vi "AcidClean.vi"() -> ()   [LabVIEW 2019]
uses:
  <vilib>/NI/Current Value Table/Type Defs/Single Tag.ctl
  <vilib>/NI/Current Value Table/Type Defs/Data Types.ctl
  <vilib>/Utility/miscctls.llb/LVPointTypeDef.ctl
  <vilib>/NI/STM/TCP/Read Meta Data (TCP Ref).vi
  <vilib>/NI/STM/TCP/Get Connection Reference (TCP).vi
  <vilib>/NI/AMC/Read Termination Message.vi
  <vilib>/NI/AMC/Create Single Message.vi
  <vilib>/NI/AMC/Update Message Routing Info.vi
  <vilib>/NI/STM/TCP/Read Meta Data (TCP Clst).vi
  <vilib>/NI/AMC/Globals.vi
  <vilib>/NI/STM/TCP/Write Message (TCP).vi
  <vilib>/NI/AMC/Send Message.vi
  <vilib>/NI/AMC/AMC.lvlib
  <vilib>/NI/STM/NI STM.lvlib
  <vilib>/NI/Current Value Table/Current Value Table.lvlib
panel:
  in  "AcidT3 Cntrl T Last Hr":bool
  out "Cleaner Control Temperature":dbl(slide) scale=0.0..60.0
  in  "Level Setpoint":dbl(knob)=40.0 min=40.0 max=85.0 step=0.5 scale=40.0..85.0
  in  "Enable Auto Fill":bool
  in  "AcidT3 Flow Last Hr":bool
  in  "AcidT3 Lev Last Hr":bool
  in  "AcidT3 T Last Hr":bool
  in  "Temperature Setpoint":dbl(knob)=25.0 min=20.0 max=60.0 step=0.5 scale=20.0..60.0
  in  "Enable Heat":bool
  out "Heater 2":bool
  out "Boolean 4":bool
  out "Boolean 2":bool
  out "Boolean 5":bool
  out "Drain":bool
  out "SuckPipe 2":bool
  out "Main Pump":bool
  in  "Tab Control":enum32{"Page 1", "ENG"}(tab)
  out "Heater Enabled":bool
  out "Amps":dbl format="%#.2g"
  out "Volts":dbl format="%#.1f"
  out "VFD T":dbl format="%#.2g"
  out "RPM":dbl format="%#.0f"
  out "Fault Code":dbl format="%#.2g"
  out "Freq":dbl format="%#.2g"
  in  "Drain Acid Clean":bool
  out "Level (L)":dbl(slide) scale=0.0..100.0
  in  "Specific Gravity":dbl(knob)=1.0 min=1.0 max=1.3 step=0.0025 scale=1.0..1.3
  out "E Stop":bool
  out "Run Enabled?":bool
  out "Cleaner Tank Temperature":dbl(slide) scale=0.0..60.0
  in  "Flow Setpoint":dbl(knob)=25.0 min=25.0 max=100.0 step=1.0 scale=25.0..100.0
  in  "Enable Clean":bool
  out "Flow rate":dbl(knob) scale=0.0..100.0
  in  "Machine":bool
  in  "Basement 4":bool
  in  "Dryer":bool
  in  "Rinse 4":bool
  in  "Rinse 3":bool
  in  "Rinse 2":bool
  in  "Basement 3":bool
  in  "Basement 2":bool
  in  "Basement 1":bool
  in  "Plater 6":bool
  in  "Plater 5":bool
  in  "Plater 4":bool
  in  "Plater 3":bool
  in  "Plater 2":bool
  in  "Plater 1":bool
  in  "Predip":bool
  in  "Rinse 1":bool
  in  "Cleaner":bool
  in  "Etch":bool
  out "status":string
  # "Module Selection"
  # "L/min"
  # "°C"
  # "°C"
  # "Motor Parameters"
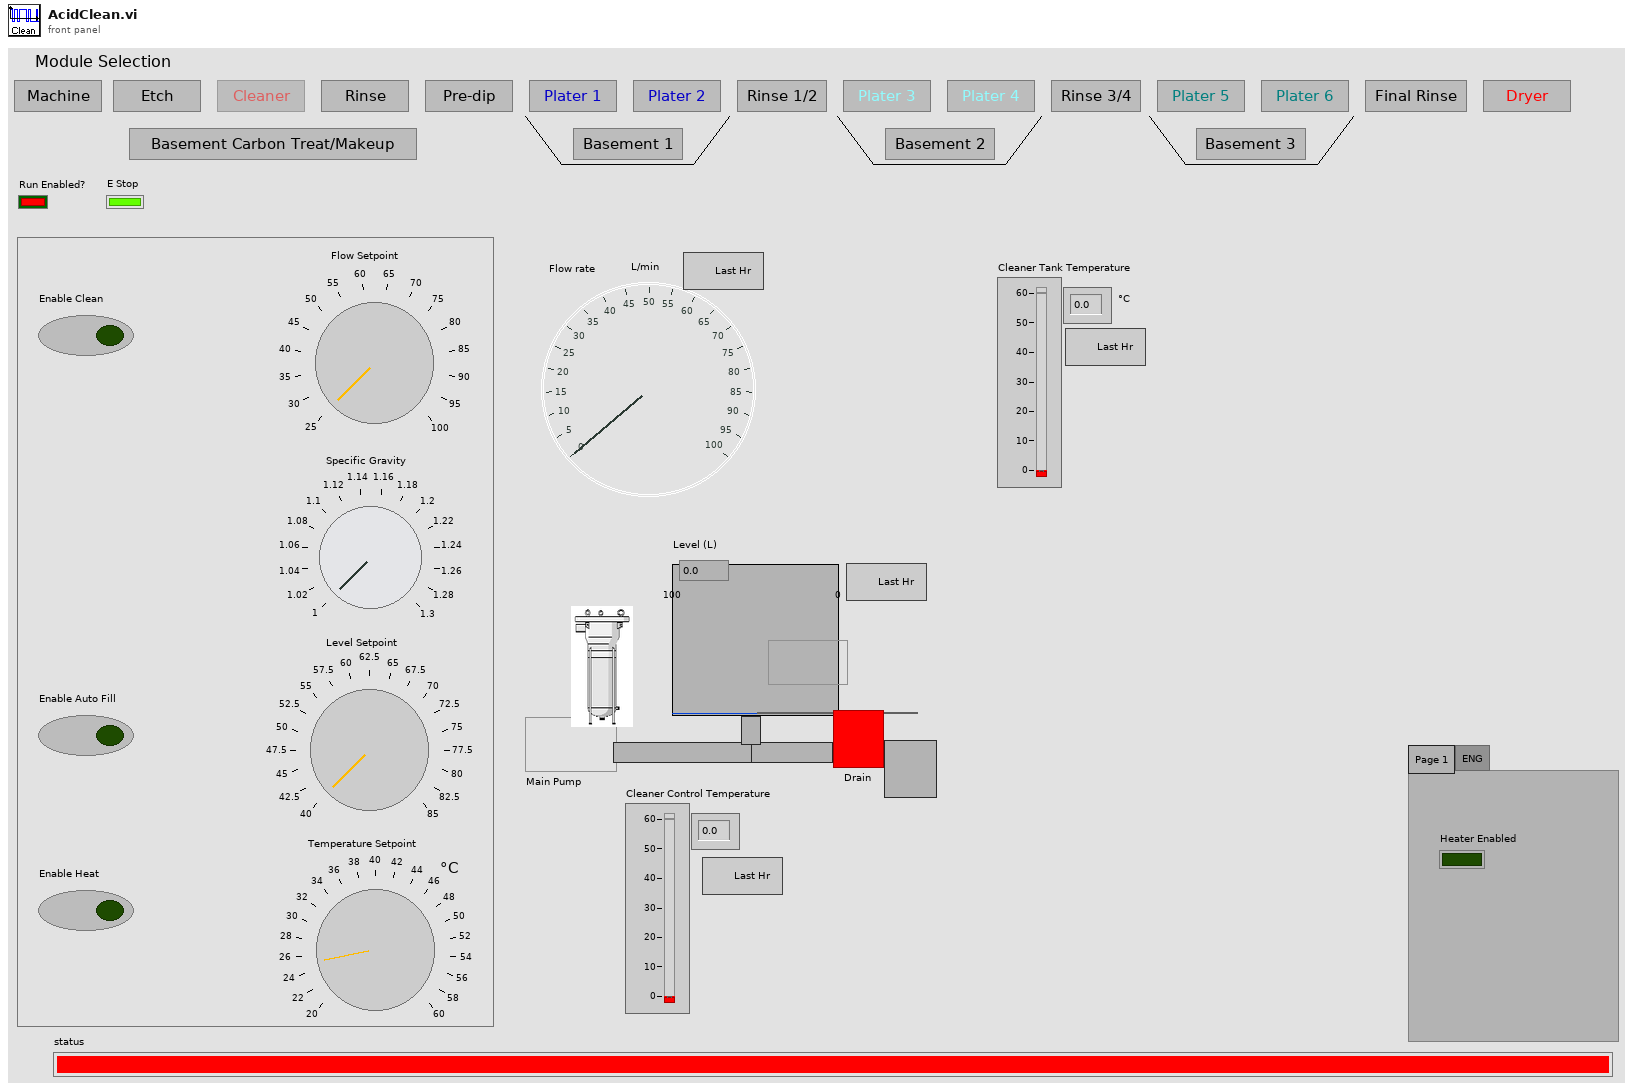
[diagram p1: front panel]
types:
  T1 = typedef "Current Value Table.lvlib/Single Tag.ctl" = cluster{"Data Type":T2, "Name":string, "Value":string, "Description":string}
  T2 = typedef "Current Value Table.lvlib/Data Types.ctl" = enum16{"Double", "Single", "I64", "I32", "I16", "I8", "U64", "U32", "U16", "U8", "String", "Boolean", "Array of U8", "Array of U16", "Array of U32", "Array of U64", "Array of I64", "Array of I32", "Array of I16", "Array of I8", "Array of Double", "Array of Single", "Array of Boolean", "Array of String"}
  T3 = typedef "NI STM.lvlib/TCP Connection Info.ctl" = cluster{"connection ID":refnum<k5>, "meta data":T4[]}
  T4 = typedef "NI STM.lvlib/MetaDataElement.ctl" = string
  T5 = typedef "AMC.lvlib/Message Queue.ctl" = refnum<queue>
  T6 = cluster{"Shift":bool, "Ctrl":bool, "Alt":bool, "Cmd":bool, "Opt":bool}
  T7 = typedef "LVPointTypeDef.ctl" = cluster{"Horizontal":i16, "Vertical":i16}
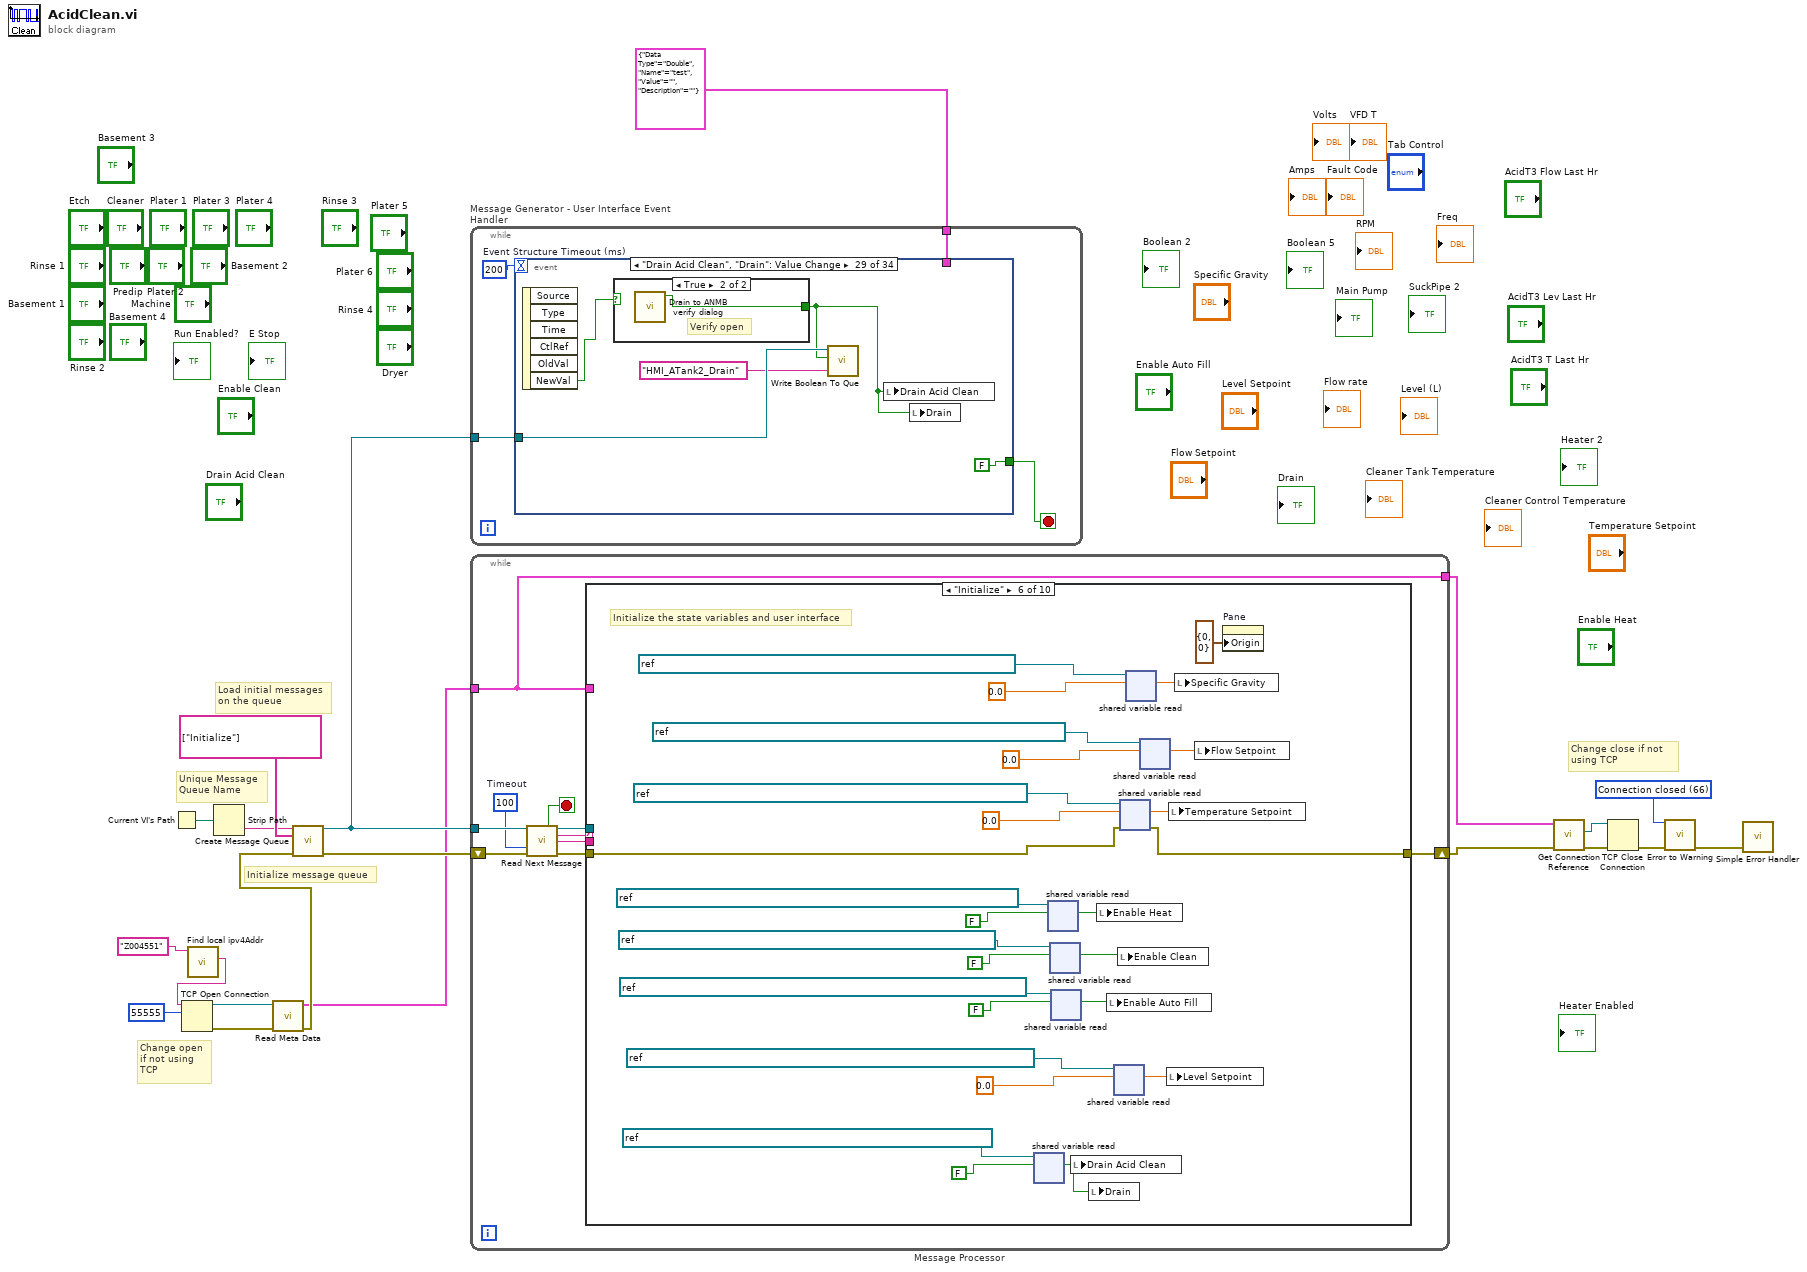
[diagram p0: block diagram]
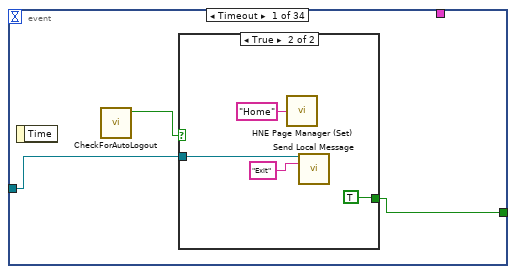
[diagram p2: hidden frame]
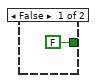
[diagram p3: hidden frame]
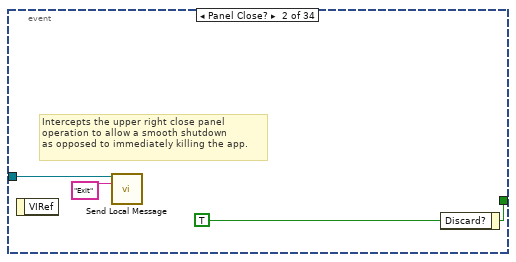
[diagram p4: hidden frame]
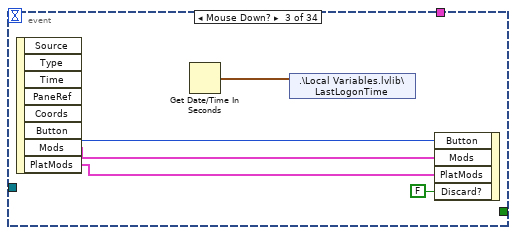
[diagram p5: hidden frame]
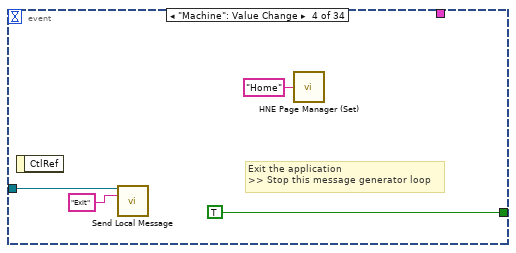
[diagram p6: hidden frame]
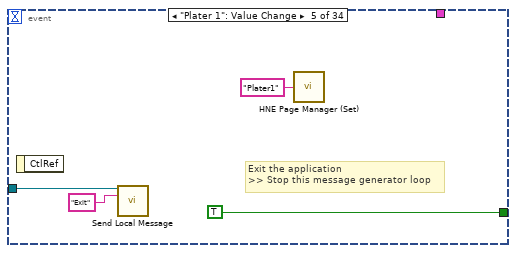
[diagram p7: hidden frame]
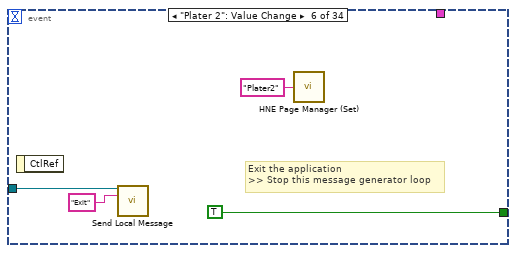
[diagram p8: hidden frame]
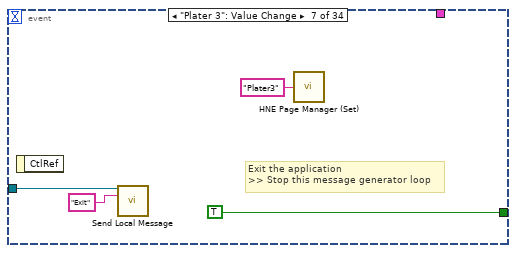
[diagram p9: hidden frame]
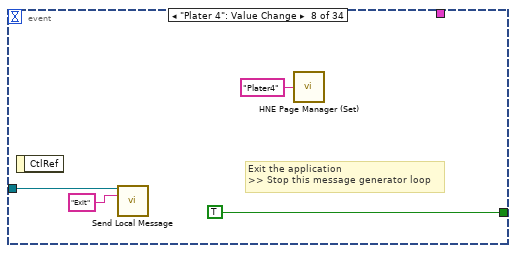
[diagram p10: hidden frame]
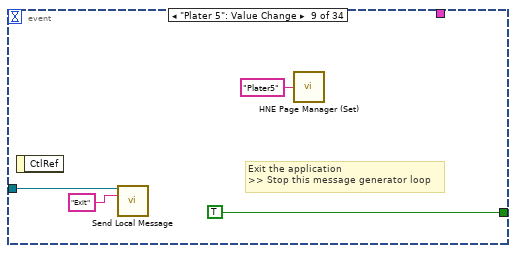
[diagram p11: hidden frame]
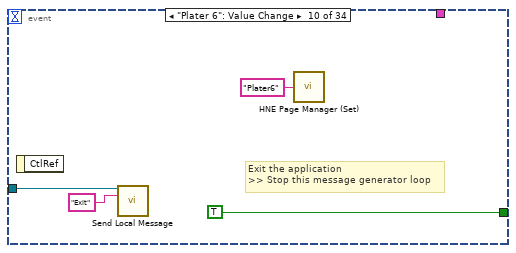
[diagram p12: hidden frame]
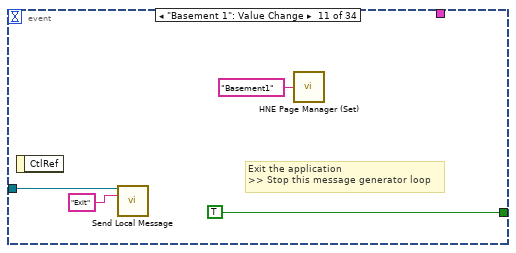
[diagram p13: hidden frame]
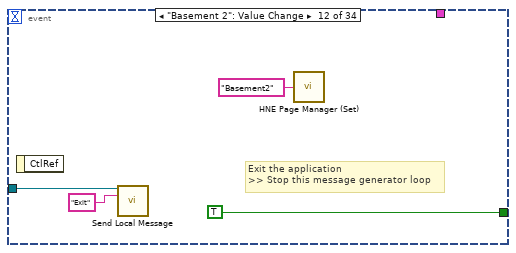
[diagram p14: hidden frame]
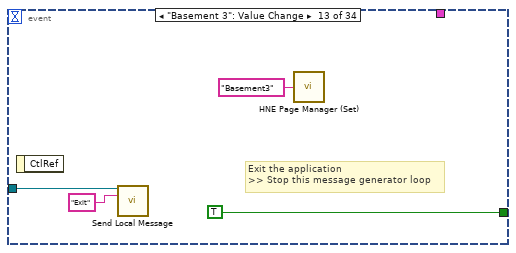
[diagram p15: hidden frame]
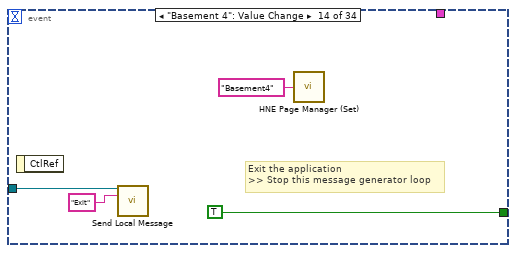
[diagram p16: hidden frame]
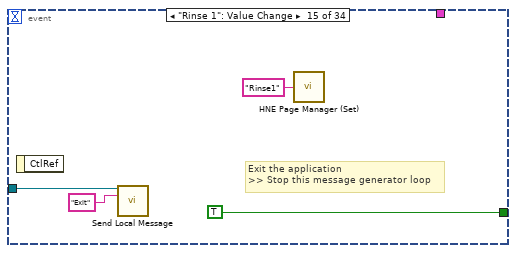
[diagram p17: hidden frame]
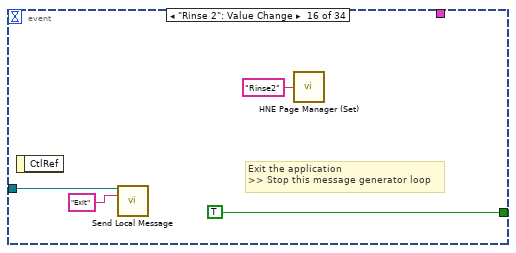
[diagram p18: hidden frame]
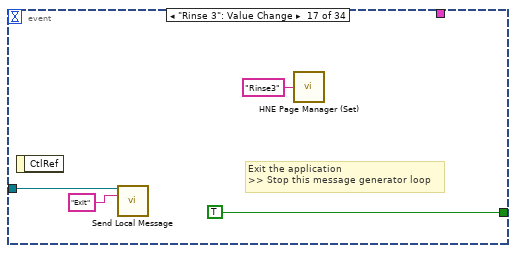
[diagram p19: hidden frame]
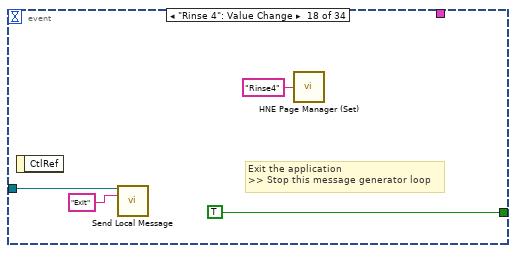
[diagram p20: hidden frame]
diagram:
  w9 = 66 items=["No Error", "Argument Error", "Memory Full", "Out of Zone", "End of File", "File Already Open", "Generic File IO Error", "File Not Found", "File Permission Error", "Disk Full", "Duplicate Path", "Too Many Files Open", "Not Enabled", "Resource File Not Found", "Cannot Add Resource", "Resource Not Found", "Image Not Found", "Image Memory Error", "Pen Does Not Exist", "Config Bad Type", "Config Token Not Found", "Config Parse Error", "Config Memory Error", "Bad External Code Format", "Bad External Code Offset", "External Code Not Present", "Null Window", "Destroy Window Mixup", "Null Menu", "Print Aborted", "Bad Print Record", "Print Driver Error", "Windows Error During Print", "Memory Error During Print", "Print Dialog Error", "Generic Print Error", "Invalid Device Refnum", "Device Not Found", "Device Parameter Error", "Device Unit Error", "Can't Open Device", "Device Call Aborted", "Generic Error", "Cancelled By User", "Object ID Too Low", "Object ID Too High", "Object Not In Heap", "Unknown Heap", "Bad DefProc ID", "DefProc Not In Table", "Message Out Of Range", "Null Method", "Unknown Message", "Manager Call Not Supported", "Bad address", "Connection In progress", "Connection timed out", "Connection is already in progress", "Network attribute not supported", "Network error", "Address in use", "System out of memory", "Connection aborted", "Connection refused", "Connection is not connected", "Connection is already connected", "Connection closed", "Initialize error (interapplication manager)", "Bad occurrence", "Wait on unbound occurrence handler", "Occurrence queue overflow", "Bad path", "Semaphore not signaled", "Unrecognized type (interapplication manager)"] ("1st Error to Convert")
  # "Change close if not using TCP"
  # "Change open if not using TCP"
  # "Initialize message queue"
  # "Unique Message\nQueue Name"
  # "Load initial messages\non the queue"
  n1 = Current VI's Path() -> (path=w16:path)
  n2 = call "Find local ipv4Addr.vi"("MachineToFind"="Z004551" ("Target IP Address")) -> ("name"=w2:string)  [unwired: 9 in, 1 out]
  n3 = TCP Open Connection(address=w2, remote port or service name=u16 55555 ("remote port")) -> (connection ID=w14:refnum<k5>, error out=w13:errorcluster)  [unwired: 1 in, 2 out]
  n4 = Strip Path(path=w16) -> (name=w19:string)  [unwired: 1 out]
  n5 = call-poly <vilib>:"Read Meta Data.vi"("error in"=w13, "connection ID"=w14) -> ("error out"=w12:errorcluster, "connection info out"=w11:T3)  [unwired: 7 in, 1 out]
  n6 = call <vilib>:"Create Message Queue.vi"("message queue name"=w19, "initial message names"=string[] ["Initialize"], "error in"=w12) -> ("message queue out"=w18:T5, "error out"=w17:errorcluster)  [unwired: 11 in]
  n7 = while "Message Generator - User Interface Event Handler" {
    tunnel: w18 -> [w22]
    tunnel: T1 {"Data Type"=enum."Double", "Name"="test", "Value"="", "Description"=""} ("Tag") -> [w21]
    stop <- w23 stop-if-true
    w24 = 200  # Event Structure Timeout (ms)
    n8 = event shown="[28] \"Drain Acid Clean\", \"Drain\": Value Change" {
      selector: _ -> [_ _ _ _ _ _ _ _ _ _ _ _ _ _ _ _ _ _ _ _ _ _ _ _ _ _ _ _ _ _ _ _ _ _]
      dyn-events: _ -> [_ _ _ _ _ _ _ _ _ _ _ _ _ _ _ _ _ _ _ _ _ _ _ _ _ _ _ _ _ _ _ _ _ _]
      timeout: w24 -> [_ _ _ _ _ _ _ _ _ _ _ _ _ _ _ _ _ _ _ _ _ _ _ _ _ _ _ _ _ _ _ _ _ _]
      tunnel: [w25 w35 _ TRUE ("Discard?") TRUE ("Discard?") TRUE ("Discard?") TRUE ("Discard?") TRUE ("Discard?") TRUE ("Discard?") TRUE ("Discard?") TRUE ("Discard?") TRUE ("Discard?") TRUE ("Discard?") TRUE ("Discard?") TRUE ("Discard?") TRUE ("Discard?") TRUE ("Discard?") TRUE ("Discard?") TRUE ("Discard?") TRUE ("Discard?") TRUE ("Discard?") FALSE ("Discard?") FALSE ("Discard?") FALSE ("Discard?") _ _ _ _ FALSE ("Discard?") FALSE ("Discard?") FALSE ("Discard?") FALSE ("Discard?") FALSE ("Discard?") _] -> w23
      tunnel: w22 -> [w26 w33 _ w42 w46 w50 w54 w58 w62 w66 w70 w74 w78 w82 w86 w90 w94 w98 w102 w106 w110 w121 w132 w143 w146 w151 w156 w161 w169 w180 w190 w200 w210 w213]
      tunnel: w21 -> [_ _ _ _ _ _ _ _ _ _ _ _ _ _ _ _ _ _ _ _ _ w115 w126 w137 _ _ _ _ _ w176 w186 w196 w206 _]
      event Timeout {
        n9 = event-data() -> ()  [unwired: 2 out]
        n10 = call "CheckForAutoLogout.vi"() -> ("Boolean"=w27:bool)  [unwired: 11 in]
        n11 = case shown="True" w27 {
          tunnel: [FALSE ("Discard?") TRUE ("Discard?")] -> w25
          tunnel: w26 -> [_ w29]
          frame False {
          }
          frame True {
            n12 = call <userlib>:"HNE Page Manager (Set).vi"("Next Page"="Home") -> ()  [unwired: 4 in, 1 out]
            n13 = call <vilib>:"Send Local Message.vi"("message queue in"=w29, "message name"="Exit") -> ()  [unwired: 11 in, 3 out]
          }
        }
      }
      event Panel Close? {
        w35 = TRUE ("Discard?")
        # "Intercepts the upper right close panel\noperation to allow a smooth shutdown\nas opposed to immediately killing the app."
        n14 = event-data() -> ()  [unwired: 2 out]
        n15 = call <vilib>:"Send Local Message.vi"("message queue in"=w33, "message name"="Exit") -> ()  [unwired: 11 in, 3 out]
        n16 = event-data("Discard?"=w35) -> ()  [unwired: 1 in, 1 out]
      }
      event Mouse Down? {
        n17 = event-data() -> ("Button"=w39:u16, "Mods"=w38:cluster{"Double Click":bool, "Menu Key":bool}, "PlatMods"=w37:T6)  [unwired: 6 out]
        n18 = Get Date/Time In Seconds() -> (seconds since 1Jan1904=w36:timestamp)
        n19 = shared-variable ".\\Local Variables.lvlib\\LastLogonTime"(w36) -> ()  [unwired: 1 in, 1 out]
        n20 = event-data("Button"=w39, "Mods"=w38, "PlatMods"=w37, "Discard?"=FALSE) -> ()  [unwired: 1 in, 1 out]
      }
      event "Machine": Value Change {
        # "Exit the application\n>> Stop this message generator loop"
        n21 = event-data() -> ()  [unwired: 2 out]
        n22 = call <vilib>:"Send Local Message.vi"("message queue in"=w42, "message name"="Exit") -> ()  [unwired: 11 in, 3 out]
        n23 = call <userlib>:"HNE Page Manager (Set).vi"("Next Page"="Home") -> ()  [unwired: 4 in, 1 out]
      }
      event "Plater 1": Value Change {
        # "Exit the application\n>> Stop this message generator loop"
        n24 = event-data() -> ()  [unwired: 2 out]
        n25 = call <vilib>:"Send Local Message.vi"("message queue in"=w46, "message name"="Exit") -> ()  [unwired: 11 in, 3 out]
        n26 = call <userlib>:"HNE Page Manager (Set).vi"("Next Page"="Plater1") -> ()  [unwired: 4 in, 1 out]
      }
      event "Plater 2": Value Change {
        # "Exit the application\n>> Stop this message generator loop"
        n27 = event-data() -> ()  [unwired: 2 out]
        n28 = call <vilib>:"Send Local Message.vi"("message queue in"=w50, "message name"="Exit") -> ()  [unwired: 11 in, 3 out]
        n29 = call <userlib>:"HNE Page Manager (Set).vi"("Next Page"="Plater2") -> ()  [unwired: 4 in, 1 out]
      }
      event "Plater 3": Value Change {
        # "Exit the application\n>> Stop this message generator loop"
        n30 = event-data() -> ()  [unwired: 2 out]
        n31 = call <vilib>:"Send Local Message.vi"("message queue in"=w54, "message name"="Exit") -> ()  [unwired: 11 in, 3 out]
        n32 = call <userlib>:"HNE Page Manager (Set).vi"("Next Page"="Plater3") -> ()  [unwired: 4 in, 1 out]
      }
      event "Plater 4": Value Change {
        # "Exit the application\n>> Stop this message generator loop"
        n33 = event-data() -> ()  [unwired: 2 out]
        n34 = call <vilib>:"Send Local Message.vi"("message queue in"=w58, "message name"="Exit") -> ()  [unwired: 11 in, 3 out]
        n35 = call <userlib>:"HNE Page Manager (Set).vi"("Next Page"="Plater4") -> ()  [unwired: 4 in, 1 out]
      }
      event "Plater 5": Value Change {
        # "Exit the application\n>> Stop this message generator loop"
        n36 = event-data() -> ()  [unwired: 2 out]
        n37 = call <vilib>:"Send Local Message.vi"("message queue in"=w62, "message name"="Exit") -> ()  [unwired: 11 in, 3 out]
        n38 = call <userlib>:"HNE Page Manager (Set).vi"("Next Page"="Plater5") -> ()  [unwired: 4 in, 1 out]
      }
      event "Plater 6": Value Change {
        # "Exit the application\n>> Stop this message generator loop"
        n39 = event-data() -> ()  [unwired: 2 out]
        n40 = call <vilib>:"Send Local Message.vi"("message queue in"=w66, "message name"="Exit") -> ()  [unwired: 11 in, 3 out]
        n41 = call <userlib>:"HNE Page Manager (Set).vi"("Next Page"="Plater6") -> ()  [unwired: 4 in, 1 out]
      }
      event "Basement 1": Value Change {
        # "Exit the application\n>> Stop this message generator loop"
        n42 = event-data() -> ()  [unwired: 2 out]
        n43 = call <vilib>:"Send Local Message.vi"("message queue in"=w70, "message name"="Exit") -> ()  [unwired: 11 in, 3 out]
        n44 = call <userlib>:"HNE Page Manager (Set).vi"("Next Page"="Basement1") -> ()  [unwired: 4 in, 1 out]
      }
      event "Basement 2": Value Change {
        # "Exit the application\n>> Stop this message generator loop"
        n45 = event-data() -> ()  [unwired: 2 out]
        n46 = call <vilib>:"Send Local Message.vi"("message queue in"=w74, "message name"="Exit") -> ()  [unwired: 11 in, 3 out]
        n47 = call <userlib>:"HNE Page Manager (Set).vi"("Next Page"="Basement2") -> ()  [unwired: 4 in, 1 out]
      }
      event "Basement 3": Value Change {
        # "Exit the application\n>> Stop this message generator loop"
        n48 = event-data() -> ()  [unwired: 2 out]
        n49 = call <vilib>:"Send Local Message.vi"("message queue in"=w78, "message name"="Exit") -> ()  [unwired: 11 in, 3 out]
        n50 = call <userlib>:"HNE Page Manager (Set).vi"("Next Page"="Basement3") -> ()  [unwired: 4 in, 1 out]
      }
      event "Basement 4": Value Change {
        # "Exit the application\n>> Stop this message generator loop"
        n51 = event-data() -> ()  [unwired: 2 out]
        n52 = call <vilib>:"Send Local Message.vi"("message queue in"=w82, "message name"="Exit") -> ()  [unwired: 11 in, 3 out]
        n53 = call <userlib>:"HNE Page Manager (Set).vi"("Next Page"="Basement4") -> ()  [unwired: 4 in, 1 out]
      }
      event "Rinse 1": Value Change {
        # "Exit the application\n>> Stop this message generator loop"
        n54 = event-data() -> ()  [unwired: 2 out]
        n55 = call <vilib>:"Send Local Message.vi"("message queue in"=w86, "message name"="Exit") -> ()  [unwired: 11 in, 3 out]
        n56 = call <userlib>:"HNE Page Manager (Set).vi"("Next Page"="Rinse1") -> ()  [unwired: 4 in, 1 out]
      }
      event "Rinse 2": Value Change {
        # "Exit the application\n>> Stop this message generator loop"
        n57 = event-data() -> ()  [unwired: 2 out]
        n58 = call <vilib>:"Send Local Message.vi"("message queue in"=w90, "message name"="Exit") -> ()  [unwired: 11 in, 3 out]
        n59 = call <userlib>:"HNE Page Manager (Set).vi"("Next Page"="Rinse2") -> ()  [unwired: 4 in, 1 out]
      }
      event "Rinse 3": Value Change {
        # "Exit the application\n>> Stop this message generator loop"
        n60 = event-data() -> ()  [unwired: 2 out]
        n61 = call <vilib>:"Send Local Message.vi"("message queue in"=w94, "message name"="Exit") -> ()  [unwired: 11 in, 3 out]
        n62 = call <userlib>:"HNE Page Manager (Set).vi"("Next Page"="Rinse3") -> ()  [unwired: 4 in, 1 out]
      }
      event "Rinse 4": Value Change {
        # "Exit the application\n>> Stop this message generator loop"
        n63 = event-data() -> ()  [unwired: 2 out]
        n64 = call <vilib>:"Send Local Message.vi"("message queue in"=w98, "message name"="Exit") -> ()  [unwired: 11 in, 3 out]
        n65 = call <userlib>:"HNE Page Manager (Set).vi"("Next Page"="Rinse4") -> ()  [unwired: 4 in, 1 out]
      }
      event "Predip": Value Change {
        # "Exit the application\n>> Stop this message generator loop"
        n66 = event-data() -> ()  [unwired: 2 out]
        n67 = call <vilib>:"Send Local Message.vi"("message queue in"=w102, "message name"="Exit") -> ()  [unwired: 11 in, 3 out]
        n68 = call <userlib>:"HNE Page Manager (Set).vi"("Next Page"="Predip") -> ()  [unwired: 4 in, 1 out]
      }
      event "Etch": Value Change {
        # "Exit the application\n>> Stop this message generator loop"
        n69 = event-data() -> ()  [unwired: 2 out]
        n70 = call <vilib>:"Send Local Message.vi"("message queue in"=w106, "message name"="Exit") -> ()  [unwired: 11 in, 3 out]
        n71 = call <userlib>:"HNE Page Manager (Set).vi"("Next Page"="Etch") -> ()  [unwired: 4 in, 1 out]
      }
      event "Dryer": Value Change {
        # "Exit the application\n>> Stop this message generator loop"
        n72 = event-data() -> ()  [unwired: 2 out]
        n73 = call <vilib>:"Send Local Message.vi"("message queue in"=w110, "message name"="Exit") -> ()  [unwired: 11 in, 3 out]
        n74 = call <userlib>:"HNE Page Manager (Set).vi"("Next Page"="Dryer") -> ()  [unwired: 4 in, 1 out]
      }
      event "Enable Clean": Value Change {
        n75 = event-data() -> ("NewVal"=w120:bool)  [unwired: 6 out]
        n76 = Boolean To (0,1)(Boolean=w120) -> (0, 1=w119:i16)
        n77 = Number To Decimal String(number=w119) -> (decimal integer string=w114:string)  [unwired: 1 in]
        n78 = Bundle By Name(cluster=w115, "Data Type"=Data_Types."Boolean", "Name"="HMI_ATank2_Enable", "Value"=w114) -> (w116:T1)
        n79 = Flatten To String(anything=w116) -> (data string=w113:string)  [unwired: 3 in, 2 out]
        n80 = call <vilib>:"Send Local Message.vi"("message queue in"=w121, "message name"="Write_Tag", "message value"=w113) -> ()  [unwired: 10 in, 3 out]
      }
      event "Enable Heat": Value Change {
        n81 = event-data() -> ("NewVal"=w131:bool)  [unwired: 6 out]
        n82 = Boolean To (0,1)(Boolean=w131) -> (0, 1=w130:i16)
        n83 = Number To Decimal String(number=w130) -> (decimal integer string=w125:string)  [unwired: 1 in]
        n84 = Bundle By Name(cluster=w126, "Data Type"=Data_Types."Boolean", "Name"="HMI_ATank2_HeatEnable", "Value"=w125) -> (w127:T1)
        n85 = Flatten To String(anything=w127) -> (data string=w124:string)  [unwired: 3 in, 2 out]
        n86 = call <vilib>:"Send Local Message.vi"("message queue in"=w132, "message name"="Write_Tag", "message value"=w124) -> ()  [unwired: 10 in, 3 out]
      }
      event "Enable Auto Fill": Value Change {
        n87 = event-data() -> ("NewVal"=w142:bool)  [unwired: 6 out]
        n88 = Boolean To (0,1)(Boolean=w142) -> (0, 1=w141:i16)
        n89 = Number To Decimal String(number=w141) -> (decimal integer string=w136:string)  [unwired: 1 in]
        n90 = Bundle By Name(cluster=w137, "Data Type"=Data_Types."Boolean", "Name"="HMI_ATank2_Fill_To_Level", "Value"=w136) -> (w138:T1)
        n91 = Flatten To String(anything=w138) -> (data string=w135:string)  [unwired: 3 in, 2 out]
        n92 = call <vilib>:"Send Local Message.vi"("message queue in"=w143, "message name"="Write_Tag", "message value"=w135) -> ()  [unwired: 10 in, 3 out]
      }
      event "AcidT3 Cntrl T Last Hr": Value Change {
        n93 = event-data() -> ("NewVal"=w147:bool)  [unwired: 6 out]
        n94 = case shown="True" w147 {
          tunnel: w146 -> [_ w150]
          frame False {
          }
          frame True {
            n95 = call <vilib>:"Send Local Message.vi"("message queue in"=w150, "message name"="DisplayLastHr", "message value"="Acid2_Temperature") -> ()  [unwired: 10 in, 3 out]
          }
        }
      }
      event "AcidT3 T Last Hr": Value Change {
        n96 = event-data() -> ("NewVal"=w152:bool)  [unwired: 6 out]
        n97 = case shown="True" w152 {
          tunnel: w151 -> [_ w155]
          frame False {
          }
          frame True {
            n98 = call <vilib>:"Send Local Message.vi"("message queue in"=w155, "message name"="DisplayLastHr", "message value"="AcidTnk2_Tank_T") -> ()  [unwired: 10 in, 3 out]
          }
        }
      }
      event "AcidT3 Lev Last Hr": Value Change {
        n99 = event-data() -> ("NewVal"=w157:bool)  [unwired: 6 out]
        n100 = case shown="True" w157 {
          tunnel: w156 -> [_ w160]
          frame False {
          }
          frame True {
            n101 = call <vilib>:"Send Local Message.vi"("message queue in"=w160, "message name"="DisplayLastHr", "message value"="Acid2_Level") -> ()  [unwired: 10 in, 3 out]
          }
        }
      }
      event "AcidT3 Flow Last Hr": Value Change {
        n102 = event-data() -> ("NewVal"=w162:bool)  [unwired: 6 out]
        n103 = case shown="True" w162 {
          tunnel: w161 -> [_ w165]
          frame False {
          }
          frame True {
            n104 = call <vilib>:"Send Local Message.vi"("message queue in"=w165, "message name"="DisplayLastHr", "message value"="Acid2_Flow") -> ()  [unwired: 10 in, 3 out]
          }
        }
      }
      event "Drain Acid Clean", "Drain": Value Change {
        n105 = event-data() -> ("NewVal"=w167:bool)  [unwired: 6 out]
        n106 = case shown="True" w167 {
          selector: w167 -> [w171 _]
          tunnel: [w171 w172] -> w166
          frame False {
            # "Always close"
          }
          frame True {
            # "Verify open"
            n107 = call "Drain to ANMB verify dialog.vi"() -> ("Drain?"=w172:bool)  [unwired: 11 in]
          }
        }
        n108 = call "Write Boolean To Que.vi"("Tag"="HMI_ATank2_Drain", "NewVal"=w166, "Queue in"=w169) -> ()  [unwired: 9 in]
        n109 = local write "Drain Acid Clean"(w166) -> ()
        n110 = local write "Drain"(w166) -> ()
      }
      event "Flow Setpoint": Value Change {
        n111 = event-data() -> ("NewVal"=w174:dbl)  [unwired: 6 out]
        n112 = Number To Fractional String(number=w174) -> (F-format string=w173:string)  [unwired: 3 in]
        n113 = Bundle By Name(cluster=w176, "Data Type"=Data_Types."Double", "Name"="HMI_ATNK2_Flow_Setpoint", "Value"=w173) -> (w177:T1)
        n114 = Flatten To String(anything=w177) -> (data string=w175:string)  [unwired: 3 in, 2 out]
        n115 = call <vilib>:"Send Local Message.vi"("message queue in"=w180, "message name"="Write_Tag", "message value"=w175) -> ()  [unwired: 10 in, 3 out]
      }
      event "Specific Gravity": Value Change {
        n116 = event-data() -> ("NewVal"=w184:dbl)  [unwired: 6 out]
        n117 = Number To Fractional String(number=w184) -> (F-format string=w183:string)  [unwired: 3 in]
        n118 = Bundle By Name(cluster=w186, "Data Type"=Data_Types."Double", "Name"="HMI_Acid2_Tank_SG", "Value"=w183) -> (w187:T1)
        n119 = Flatten To String(anything=w187) -> (data string=w185:string)  [unwired: 3 in, 2 out]
        n120 = call <vilib>:"Send Local Message.vi"("message queue in"=w190, "message name"="Write_Tag", "message value"=w185) -> ()  [unwired: 10 in, 3 out]
      }
      event "Temperature Setpoint": Value Change {
        n121 = event-data() -> ("NewVal"=w194:dbl)  [unwired: 6 out]
        n122 = Number To Fractional String(number=w194) -> (F-format string=w193:string)  [unwired: 3 in]
        n123 = Bundle By Name(cluster=w196, "Data Type"=Data_Types."Double", "Name"="HMI_ATNK2_T_Setpoint", "Value"=w193) -> (w197:T1)
        n124 = Flatten To String(anything=w197) -> (data string=w195:string)  [unwired: 3 in, 2 out]
        n125 = call <vilib>:"Send Local Message.vi"("message queue in"=w200, "message name"="Write_Tag", "message value"=w195) -> ()  [unwired: 10 in, 3 out]
      }
      event "Level Setpoint": Value Change {
        n126 = event-data() -> ("NewVal"=w204:dbl)  [unwired: 6 out]
        n127 = Number To Fractional String(number=w204) -> (F-format string=w203:string)  [unwired: 3 in]
        n128 = Bundle By Name(cluster=w206, "Data Type"=Data_Types."Double", "Name"="HMI_ATank2_Level_SetPnt", "Value"=w203) -> (w207:T1)
        n129 = Flatten To String(anything=w207) -> (data string=w205:string)  [unwired: 3 in, 2 out]
        n130 = call <vilib>:"Send Local Message.vi"("message queue in"=w210, "message name"="Write_Tag", "message value"=w205) -> ()  [unwired: 10 in, 3 out]
      }
      event Menu Selection (User) {
        # "Add run-time menu items to the message\nqueue. The message handler case names must match the menu ItemTag names."
        n131 = event-data() -> ("ItemTag"=w214:string)  [unwired: 1 out]
        n132 = call <vilib>:"Send Local Message.vi"("message queue in"=w213, "message name"=w214) -> ()  [unwired: 11 in, 3 out]
      }
    }
  }
  n133 = while "Message Processor" {
    shift-left: w17 -> [w220]
    shift-right: [w224] -> w4
    tunnel: w18 -> [w221]
    tunnel: w11 -> [w215]
    tunnel: [w215] -> w5
    stop <- w223 stop-if-true
    w216 = 100  # Timeout
    n134 = call <vilib>:"Read Next Message.vi"("message queue in"=w221, "timeout (1 ms)"=w216, "error in"=w220) -> ("exit process?"=w223:bool, "message queue out"=w222:T5, "message name"=w218:string, "message value"=w217:string, "error out"=w219:errorcluster)  [unwired: 5 in, 3 out]
    n135 = case shown="\"Initialize\"" w218 {
      selector: w218 -> [_ _ w233 _ _ _ _ _ _ _]
      tunnel: w222 -> [_ _ _ _ _ _ w266 _ _ _]
      tunnel: w219 -> [w225 w230 w234 w235 w237 w250 w267 w269 w273 w275]
      tunnel: [w225 w230 w234 errorcluster {"status"=FALSE, "code"=0, "source"=""} ("error out") w237 w249 w265 w269 w272 w275] -> w224
      tunnel: w217 -> [_ _ _ _ _ _ _ _ w270 w276]
      tunnel: w215 -> [_ _ _ _ _ _ _ _ w271 _]
      frame "---------- Framework Operations ----------" {
        # "Dummy case to add a seperator in the Case Structure menu"
      }
      frame "", "Idle" {
        # "Idle Case - this case is called after a Timeout on the Get Next Message from Queue VI, if no new messages are present on the queue. This case can be used for housekeeping tasks such as updating the UI."
        n136 = control-ref of="status"() -> (w229:refnum<vi>)
        n137 = local read "Main Pump"() -> (w227:bool)
        n138 = local read "Drain"() -> (w228:bool)
        n139 = call <userlib>:"TAE Format Alarm Ticker.vi"("Alarm Ticker Ref"=w229) -> ()  [unwired: 15 in]
        n140 = Or(x=w228, y=w227) -> (x .or. y?=→"Boolean 4":bool)
      }
      frame "Missing Message Handler", Default {
        # "Call this case if a message is received that is not handled \nby any other case. Typically this is a programming error\nas a result of a typo or unhandled message/missing message handler."
        n141 = Format Into String(format string="DevError: Missing message handler for '%s\" message." ("message"), w233) -> (resulting string=w231:string)  [unwired: 2 in, 1 out]
        n142 = One Button Dialog(message=w231) -> ()  [unwired: 2 out]
      }
      frame "Error" {
        # "General Error Case - this case is called if an error is passed using the error cluster below. Typically most new errors should be handed in each individual case and not passed in the rror cluster. If necessary a custom error handler case should be added and called from other cases."
        n143 = call <vilib>:"Simple Error Handler.vi"("error in (no error)"=w235) -> ()  [unwired: 1 in, 8 out]
      }
      frame "---------- Generic Operations ----------" {
        # "Dummy case to add a seperator in the Case Structure menu"
      }
      frame "Initialize" {
        # "Initialize the state variables and user interface"
        n144 = shared-variable-read(refnum<k21> "ni.var.psp://z004551/CDL0100 ReadWriteTags/HMI_ATank2_Drain" ("shared variable refnum in"), FALSE) -> (w253:bool)  [unwired: 1 in, 3 out]
        n145 = shared-variable-read(refnum<k21> "ni.var.psp://z004551/CDL0100 ReadWriteTags/HMI_ATank2_HeatEnable" ("shared variable refnum in"), FALSE) -> (w245:bool)  [unwired: 1 in, 3 out]
        n146 = shared-variable-read(refnum<k21> "ni.var.psp://z004551/CDL0100 ReadWriteTags/HMI_ATank2_Enable" ("shared variable refnum in"), FALSE) -> (w262:bool)  [unwired: 1 in, 3 out]
        n147 = shared-variable-read(refnum<k21> "ni.var.psp://z004551/CDL0100 ReadWriteTags/HMI_ATank2_Fill_To_Level" ("shared variable refnum in"), FALSE) -> (w242:bool)  [unwired: 1 in, 3 out]
        n148 = local write "Drain Acid Clean"(w253) -> ()
        n149 = local write "Drain"(w253) -> ()
        n150 = local write "Enable Heat"(w245) -> ()
        n151 = local write "Enable Auto Fill"(w242) -> ()
        n152 = shared-variable-read(refnum<k21> "ni.var.psp://z004551/CDL0100 ReadWriteTags/HMI_ATank2_Level_SetPnt" ("shared variable refnum in"), 0.0) -> (w239:dbl)  [unwired: 1 in, 3 out]
        n153 = local write "Enable Clean"(w262) -> ()
        n154 = shared-variable-read(refnum<k21> "ni.var.psp://z004551/CDL0100 ReadWriteTags/HMI_ATNK2_T_Setpoint" ("shared variable refnum in"), w250, 0.0) -> (w249:errorcluster, w248:dbl)  [unwired: 2 out]
        n155 = shared-variable-read(refnum<k21> "ni.var.psp://z004551/CDL0100 ReadWriteTags/HMI_Acid2_Tank_SG" ("shared variable refnum in"), 0.0) -> (w254:dbl)  [unwired: 1 in, 3 out]
        n156 = shared-variable-read(refnum<k21> "ni.var.psp://z004551/CDL0100 ReadWriteTags/HMI_ATNK2_Flow_Setpoint" ("shared variable refnum in"), 0.0) -> (w259:dbl)  [unwired: 1 in, 3 out]
        n157 = local write "Level Setpoint"(w239) -> ()
        n158 = local write "Temperature Setpoint"(w248) -> ()
        n159 = local write "Specific Gravity"(w254) -> ()
        n160 = local write "Flow Setpoint"(w259) -> ()
        n161 = property on="Pane" class="Pane"("Origin"=T7 {"Horizontal"=0, "Vertical"=0}) -> ()  [unwired: 2 in, 2 out]
      }
      frame "Exit" {
        # "Destroy message queue >> this will halt the UI event handler loop"
        # "Stop the VI\n>> Perform any cleanup tasks in this message case.\n>> Clear display before closing."
        n162 = call <vilib>:"Destroy Message Queue.vi"("message queue in"=w266, "error in"=w267) -> ("error out"=w265:errorcluster)  [unwired: 11 in, 2 out]
        n163 = local write "status"("" ("Status")) -> ()
      }
      frame "---------- Application Operations ----------" {
        # "Dummy case to add a seperator in the Case Structure menu"
      }
      frame "Write_Tag" {
        n164 = call-poly <vilib>:"Write Message.vi"("error in"=w273, "data"=w270, "name"="WriteTag", "connection info in"=w271) -> ("error out"=w272:errorcluster)  [unwired: 6 in, 1 out]
      }
      frame "DisplayLastHr" {
        n165 = call "Trace Variable 1 hour Popup.vi"("Tag"=w276) -> ()  [unwired: 11 in]
      }
    }
  }
  n166 = call-poly <vilib>:"Get Connection Reference.vi"("error in"=w4, "connection info in"=w5) -> ("error out"=w8:errorcluster, "connection ID out"=w7:refnum<k5>)  [unwired: 8 out]
  n167 = TCP Close Connection(connection ID=w7, error in (no error)=w8) -> (error out=w10:errorcluster)  [unwired: 2 out]
  n168 = call <vilib>:"Error to Warning.vi"("1st Error to Convert"=w9, "error in"=w10) -> ("warning out"=w6:errorcluster)  [unwired: 3 in, 10 out]
  n169 = call <vilib>:"Simple Error Handler.vi"("error in (no error)"=w6) -> ()  [unwired: 4 in, 5 out]
